vi "getMFC_ring.vi"() -> ()   [LabVIEW 2011]
uses:
  globals.vi
  MFC_ring.ctl
panel:
  out "output array":string[](array[string])
  in  "Tab Control":enum32{"Page 1", "Page 2"}(tab)
  in  "D/A Cards":T2 {"D/A (12-bit) Card"."Channel"."Channel" items=["N2 flow (NMFC1)", "H2 flow (HMFC1)", "Al flow (AlMFC1)"]; "Quad D/A (10-bit) Cards"."Channels 5"."Channel 5" items=["flow 1", "flow 2", "flow 3"]; "Quad D/A (10-bit) Cards"."Channels 5"."Channel 4" items=["flow 1", "flow 2", "flow 3"]; "Quad D/A (10-bit) Cards"."Channels 5"."Channel 3" items=["flow 1", "flow 2", "flow 3"]; "Quad D/A (10-bit) Cards"."Channels 5"."Channel 2" items=["flow 1", "flow 2", "flow 3"]; "Quad D/A (10-bit) Cards"."Channels 4"."Channel 5" items=["flow 1", "flow 2", "flow 3"]; "Quad D/A (10-bit) Cards"."Channels 4"."Channel 4" items=["flow 1", "flow 2", "flow 3"]; "Quad D/A (10-bit) Cards"."Channels 4"."Channel 3" items=["flow 1", "flow 2", "flow 3"]; "Quad D/A (10-bit) Cards"."Channels 4"."Channel 2" items=["flow 1", "flow 2", "flow 3"]; "Quad D/A (10-bit) Cards"."Channels 3"."Channel 5" items=["flow 1", "flow 2", "flow 3"]; "Quad D/A (10-bit) Cards"."Channels 3"."Channel 4" items=["flow 1", "flow 2", "flow 3"]; "Quad D/A (10-bit) Cards"."Channels 3"."Channel 3" items=["flow 1", "flow 2", "flow 3"]; "Quad D/A (10-bit) Cards"."Channels 3"."Channel 2" items=["flow 1", "flow 2", "flow 3"]; "Quad D/A (10-bit) Cards"."Channels 2"."Channel 5" items=["flow 1", "flow 2", "flow 3"]; "Quad D/A (10-bit) Cards"."Channels 2"."Channel 4" items=["flow 1", "flow 2", "flow 3"]; "Quad D/A (10-bit) Cards"."Channels 2"."Channel 3" items=["flow 1", "flow 2", "flow 3"]; "Quad D/A (10-bit) Cards"."Channels 2"."Channel 2" items=["flow 1", "flow 2", "flow 3"]; "Quad D/A (10-bit) Cards"."Channels"."Channel 5" items=["flow 1", "flow 2", "flow 3"]; "Quad D/A (10-bit) Cards"."Channels"."Channel 4" items=["flow 1", "flow 2", "flow 3"]; "Quad D/A (10-bit) Cards"."Channels"."Channel 3" items=["flow 1", "flow 2", "flow 3"]; "Quad D/A (10-bit) Cards"."Channels"."Channel 2" items=["flow 1", "flow 2", "flow 3"]}
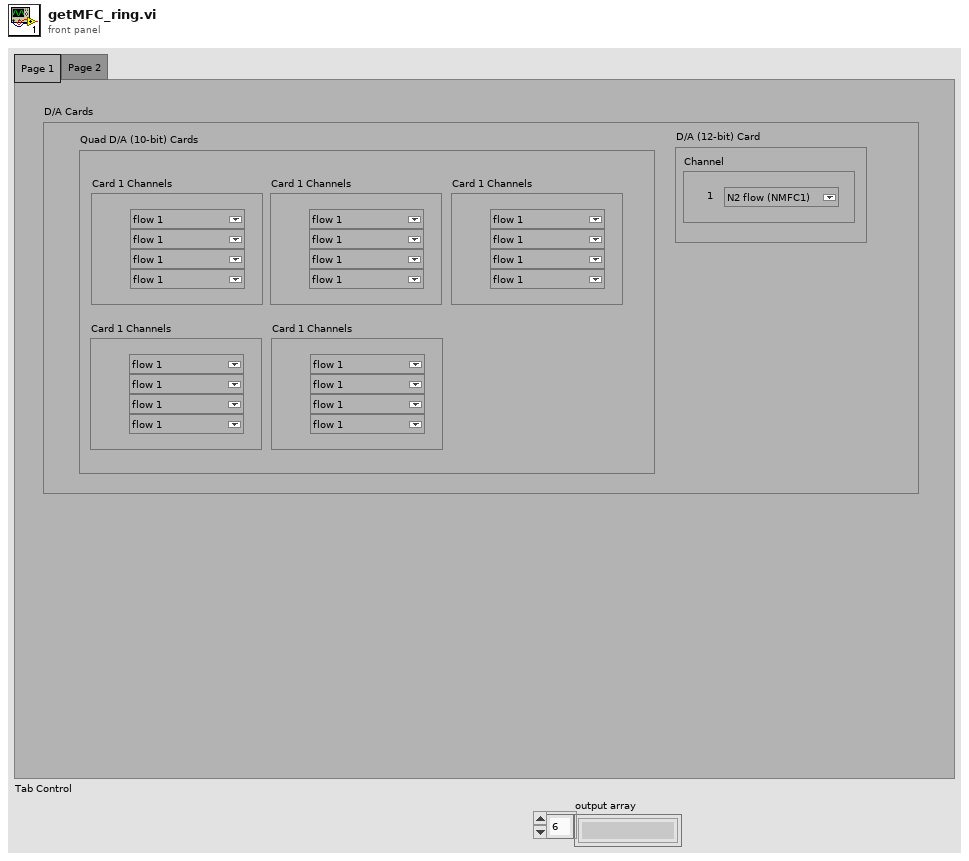
[diagram p1: front panel]
types:
  T1 = typedef "MFC_ring.ctl" = u16
  T2 = cluster{"Quad D/A (10-bit) Cards":cluster{"Channels":cluster{"Channel 2":u16, "Channel 3":u16, "Channel 4":u16, "Channel 5":u16}, "Channels 2":cluster{"Channel 2":u16, "Channel 3":u16, "Channel 4":u16, "Channel 5":u16}, "Channels 3":cluster{"Channel 2":u16, "Channel 3":u16, "Channel 4":u16, "Channel 5":u16}, "Channels 4":cluster{"Channel 2":u16, "Channel 3":u16, "Channel 4":u16, "Channel 5":u16}, "Channels 5":cluster{"Channel 2":u16, "Channel 3":u16, "Channel 4":u16, "Channel 5":u16}}, "D/A (12-bit) Card":cluster{"Channel":cluster{"Channel":T1}}}
  T3 = cluster{"NMFC1":cluster{"MFC Range":u16, "MFC Name":string}, "HMFC1":cluster{"MFC Range":u16, "MFC Name":string}, "ALMFC1":cluster{"MFC Range":u16, "MFC Name":string}, "ALMFC1 2":cluster{"MFC Range":u16, "MFC Name":string}, "ALMFC1 3":cluster{"MFC Range":u16, "MFC Name":string}, "ALMFC1 4":cluster{"MFC Range":u16, "MFC Name":string}, "ALMFC1 5":cluster{"MFC Range":u16, "MFC Name":string}}
  T4 = cluster{"Channels":cluster{"Channel 2":u16, "Channel 3":u16, "Channel 4":u16, "Channel 5":u16}, "Channels 2":cluster{"Channel 2":u16, "Channel 3":u16, "Channel 4":u16, "Channel 5":u16}, "Channels 3":cluster{"Channel 2":u16, "Channel 3":u16, "Channel 4":u16, "Channel 5":u16}, "Channels 4":cluster{"Channel 2":u16, "Channel 3":u16, "Channel 4":u16, "Channel 5":u16}, "Channels 5":cluster{"Channel 2":u16, "Channel 3":u16, "Channel 4":u16, "Channel 5":u16}}
  T5 = cluster{"Channel 2":u16, "Channel 3":u16, "Channel 4":u16, "Channel 5":u16}[]
  T6 = cluster{"Channel 2":u16, "Channel 3":u16, "Channel 4":u16, "Channel 5":u16}
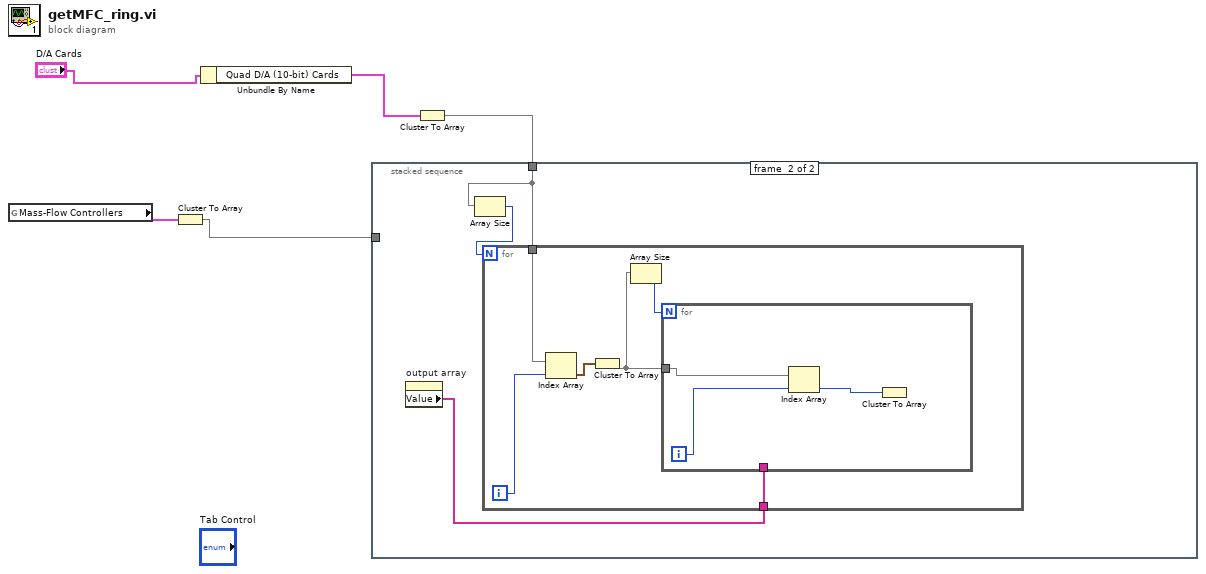
[diagram p0: block diagram]
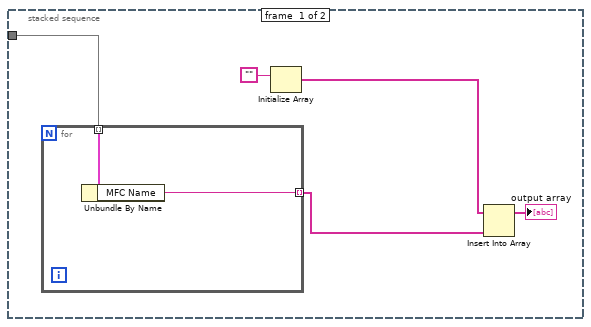
[diagram p2: hidden frame]
diagram:
  n1 = global read "globals.vi" "Mass-Flow Controllers"() -> (w5:T3)
  n2 = Cluster To Array(cluster=w5) -> (array=w4:cluster{"MFC Range":u16, "MFC Name":string}[])
  n3 = Unbundle By Name("D/A Cards") -> ("Quad D/A (10-bit) Cards"=w3:T4)
  n4 = Cluster To Array(cluster=w3) -> (array=w2:T5)
  n5 = stacked-sequence {
    tunnel: w4 -> [w7 _]
    tunnel: w2 -> [_ w14]
    frame #0 {
      n6 = for {
        tunnel: w7 -> [w12] mode=indexing
        tunnel: [w11] -> w9 mode=indexing
        n7 = Unbundle By Name(w12) -> ("MFC Name"=w11:string)
      }
      n8 = Initialize Array("") -> (w8:string[])  [unwired: 1 in]
      n9 = Insert Into Array(array=w8, new element=w9) -> (→"output array":string[])  [unwired: 1 in]
    }
    frame #1 {
      n10 = property on="output array" class="Arr (strict)"() -> ("Value"=w15:string[])  [unwired: 2 in, 2 out]
      n11 = Array Size(array=w14) -> (size(s)=w13:i32)
      n12 = for {
        N: w13 -> [_]
        tunnel: w14 -> [w20]
        tunnel: w15 -> [w21]
        i -> [w19]
        n13 = Index Array(array=w20, index=w19) -> (element=w18:T6)
        n14 = Cluster To Array(cluster=w18) -> (array=w16:u16[])
        n15 = Array Size(array=w16) -> (size(s)=w17:i32)
        n16 = for {
          N: w17 -> [_]
          tunnel: w21 -> [_]
          tunnel: w16 -> [w24]
          i -> [w23]
          n17 = Index Array(array=w24, index=w23) -> (element=w22:u16)
          n18 = Cluster To Array(cluster=w22) -> ()  [unwired: 1 out]
        }
      }
    }
  }
